vi "氨氮加标回收状态全局变量.vi"() -> ()   [LabVIEW 2016, in "质控单元.lvlib"]
panel:
  out "CODCr加标回收率":dbl caption="加标回收率" format="%.2f"
  out "CODCr加标体积":dbl caption="加标体积" format="%.3f"
  out "CODCr母液浓度":dbl caption="加标母液浓度" format="%.2f"
  out "CODCr加标水杯定容体积":dbl caption="加标水杯定容体积" format="%.2f"
  out "CODCr加标后水样浓度":dbl caption="加标后水样浓度" format="%.2f"
  out "CODCr加标前水样浓度":dbl caption="加标前水样浓度" format="%.2f"
  out "CODCr检出限":dbl caption="检出限" format="%.2f"
  out "CODCr量程":dbl caption="量程" format="%.2f"
  out "CODCr状态":u16(ring) caption="状态" items=["待机", "润洗", "进样", "等待取液", "排液"]
  out "总氮加标回收率":dbl caption="加标回收率" format="%.2f"
  out "总氮加标体积":dbl caption="加标体积" format="%.3f"
  out "总氮母液浓度":dbl caption="加标母液浓度" format="%.3f"
  out "总氮加标水杯定容体积":dbl caption="加标水杯定容体积" format="%.2f"
  out "总氮加标后水样浓度":dbl caption="加标后水样浓度" format="%.3f"
  out "总氮加标前水样浓度":dbl caption="加标前水样浓度" format="%.3f"
  out "总氮检出限":dbl caption="检出限" format="%.3f"
  out "总氮量程":dbl caption="量程" format="%.2f"
  out "总氮状态":u16(ring) caption="状态" items=["待机", "润洗", "进样", "等待取液", "排液"]
  out "CODMn加标回收率":dbl caption="加标回收率" format="%#_6f"
  out "CODMn加标体积":dbl caption="加标体积"
  out "CODMn母液浓度":dbl caption="加标母液浓度"
  out "CODMn加标水杯定容体积":dbl caption="加标水杯定容体积"
  out "CODMn加标后水样浓度":dbl caption="加标后水样浓度"
  out "CODMn加标前水样浓度":dbl caption="加标前水样浓度"
  out "CODMn检出限":dbl caption="检出限"
  out "CODMn量程":dbl caption="量程"
  out "COD状态":u16(ring) caption="状态" items=["待机", "润洗", "进样", "等待取液", "排液"]
  out "总磷加标回收率":dbl caption="加标回收率" format="%#_6f"
  out "总磷加标体积":dbl caption="加标体积"
  out "总磷母液浓度":dbl caption="加标母液浓度"
  out "总磷加标水杯定容体积":dbl caption="加标水杯定容体积"
  out "总磷加标后水样浓度":dbl caption="加标后水样浓度"
  out "总磷加标前水样浓度":dbl caption="加标前水样浓度"
  out "总磷检出限":dbl caption="检出限"
  out "总磷量程":dbl caption="量程"
  out "总磷状态":u16(ring) caption="状态" items=["待机", "润洗", "进样", "等待取液", "排液"]
  out "氨氮加标回收率":dbl caption="加标回收率" format="%#_6f"
  out "氨氮加标体积":dbl caption="加标体积"
  out "氨氮母液浓度":dbl caption="加标母液浓度"
  out "氨氮加标水杯定容体积":dbl caption="加标水杯定容体积"
  out "氨氮加标后水样浓度":dbl caption="加标后水样浓度"
  out "氨氮加标前水样浓度":dbl caption="加标前水样浓度"
  out "氨氮检出限":dbl caption="检出限"
  out "氨氮量程":dbl caption="量程"
  out "氨氮状态":u16(ring) caption="状态" items=["待机", "润洗", "进样", "等待取液", "排液"]
  # "氨氮质控参数"
  # "CODCr质控参数"
  # "%"
  # "mL"
  # "mg/L"
  # "mL"
  # "mg/L"
  # "mg/L"
  # "mg/L"
  # "mg/L"
  # "总氮质控参数"
  # "%"
  # "mL"
  # "mg/L"
  # "mL"
  # "mg/L"
  # "mg/L"
  # "mg/L"
  # "mg/L"
  # "CODMn质控参数"
  # "%"
  # "mL"
  # "mg/L"
  # "mL"
  # "mg/L"
  # "mg/L"
  # "mg/L"
  # "mg/L"
  # "总磷质控参数"
  # "%"
  # "mL"
  # "mg/L"
  # "mL"
  # "mg/L"
  # "mg/L"
  # "mg/L"
  # "mg/L"
  # "%"
  # "mL"
  # "mg/L"
  # "mL"
  # "mg/L"
  # "mg/L"
  # "mg/L"
  # "mg/L"
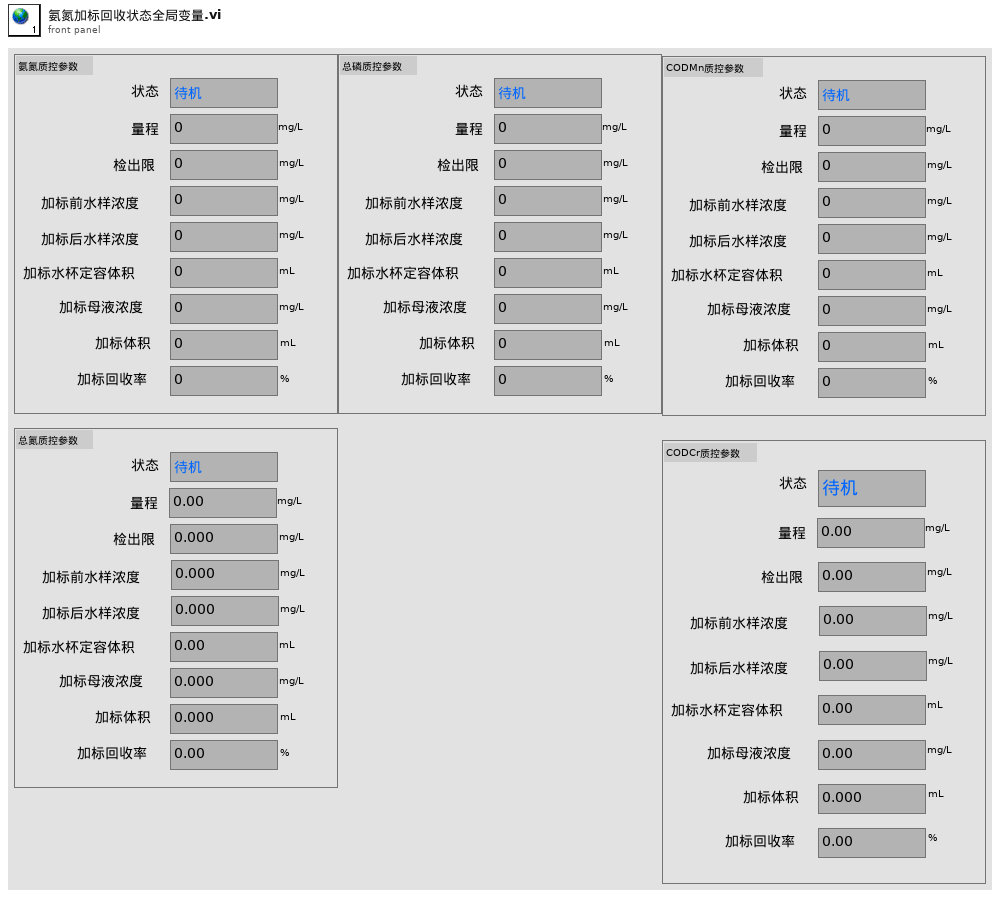
[diagram p1: front panel]
diagram:
